vi "targetVI.vi"() -> ()   [LabVIEW 2017]
uses:
  <vilib>/rvi/Emulation/niFpgaGetClockAttributes.vi
  <vilib>/rvi/Emulation/niFpgaSctlEmulationGetInTimedLoop.vi
  <vilib>/rvi/Emulation/niFpgaEmulationReportErrorSimple.vi
  <vilib>/rvi/interface/RandomDataEmulation/niFpgaRandomDataHandleErrors.vi
  <vilib>/rvi/Emulation/niFpgaCriticalErrorInLSC.vi
  <vilib>/rvi/Analysis/common/FxpNativeNode/niFpgaFxpNative.xnode
  <vilib>/rvi/DataTransferAndStorage/Container/XNode/niFpgaContainer.xnode
  <vilib>/rvi/interface/RandomDataEmulation/nirviRandomDataFpgaReadWriteTemplate.vi
panel:
  out "Timed Out?":bool
  out "Numeric":fxp<+/-,32,32>
  in  "Boolean":bool
  out "loop count":fxp<+/-,32,32>
  out "y":fxp<+/-,16,16>
  in  "end point":fxp<+/-,16,16>
  in  "start point":fxp<+/-,16,16>
  in  "update time":fxp<+,16,16> caption="update time(mSec)"
  in  "N pts in waveform":fxp<+/-,16,16>
  in  "stop":bool
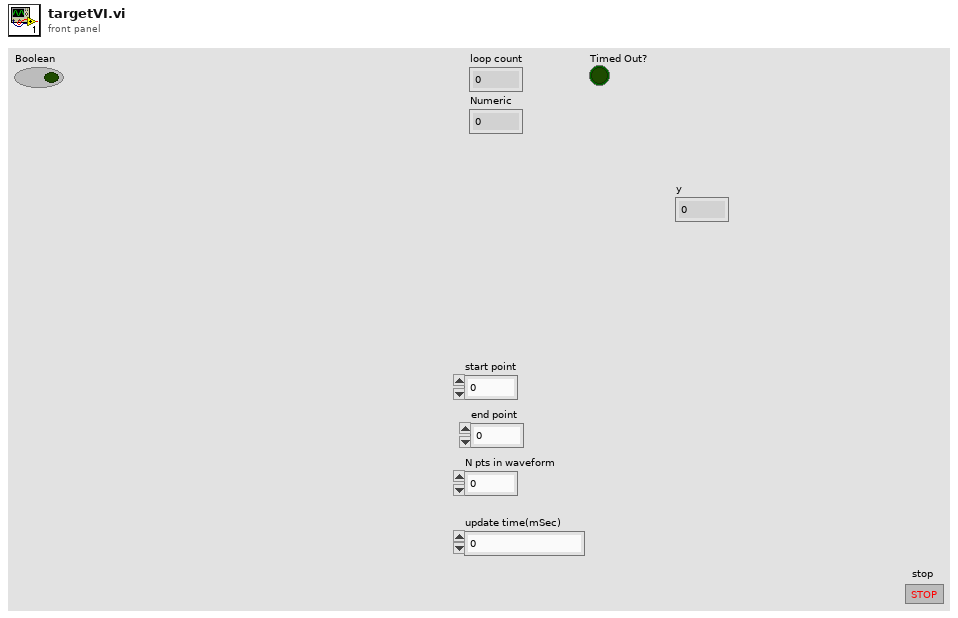
[diagram p1: front panel]
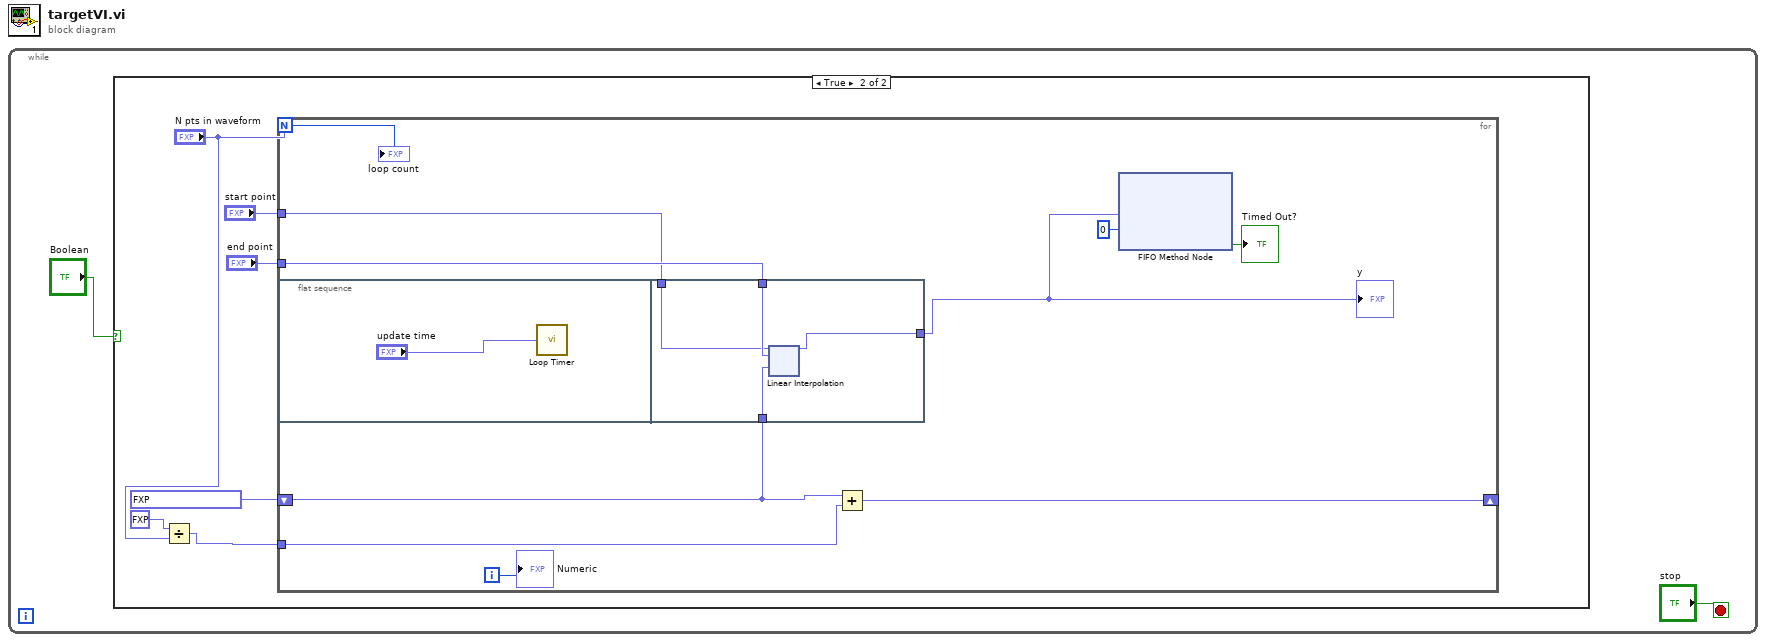
[diagram p0: block diagram]
diagram:
  n1 = while {
    stop <- "stop" stop-if-true
    n2 = case shown="True" "Boolean" {
      frame False {
      }
      frame True {
        n3 = Divide(x=fxp<+,1,1> 1.0, y="N pts in waveform") -> (x/y=w3:fxp<+/-,18,2>)
        n4 = for {
          N: "N pts in waveform" -> [w13]
          tunnel: "end point" -> [w18]
          tunnel: "start point" -> [w17]
          tunnel: w3 -> [w16]
          shift-right: [w15] -> _
          shift-left: fxp<+,16,0> 0.0 -> [w14]
          i -> [w12]
          n5 = flat-sequence {
            tunnel: w18 -> [w23]
            tunnel: w17 -> [w22]
            tunnel: [w21] -> w11
            tunnel: w14 -> [w20]
            frame #0 {
              n6 = call "Loop Timer"("Count(mSec)"="update time") -> ()  [unwired: 1 out]
            }
            frame #1 {
              n7 = xnode ("Linear Interpolation")("y0"=w22, "y1"=w23, "x"=w20) -> ("y"=w21:fxp<+/-,16,16>)
            }
          }
          n8 = Add(x=w14, y=w16) -> (x+y=w15:fxp<+,16,0>)
          n9 = xnode ("FIFO Method Node")("Element"=w11, "Timeout"=0) -> ("Timed Out?"=→"Timed Out?":bool)  [unwired: 1 in, 1 out]
          "loop count" <- w13
          "Numeric" <- w12
          "y" <- w11
        }
      }
    }
  }
